vi "4.7.vi"() -> (0 "请在1-1000猜":dbl format="%#g", 1 "循环次数":i32, 2 "随机数":i32)   [LabVIEW 2017]
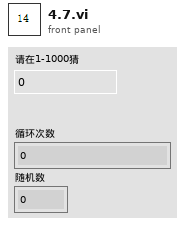
[diagram p1: front panel]
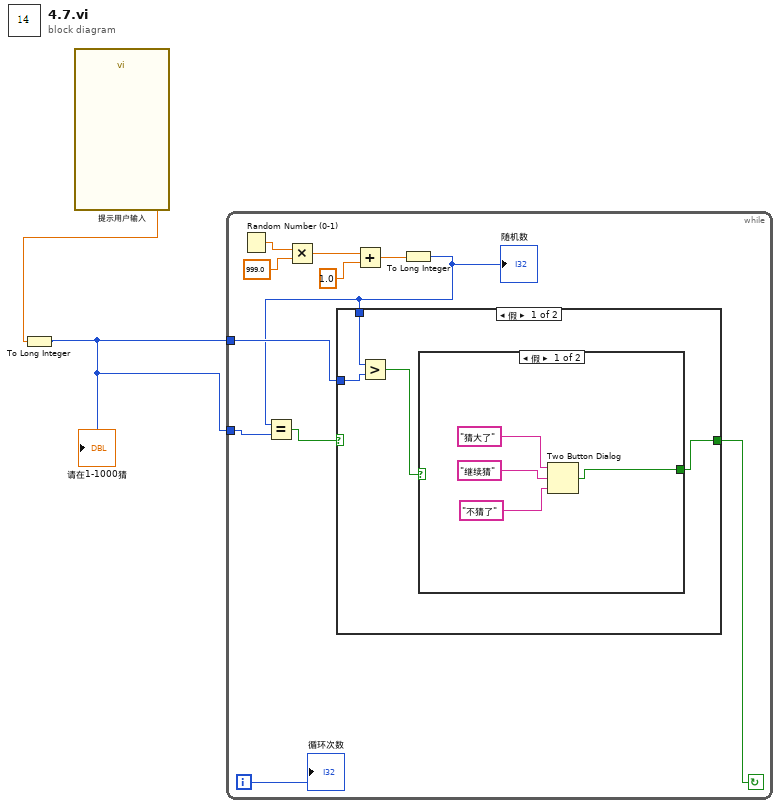
[diagram p0: block diagram]
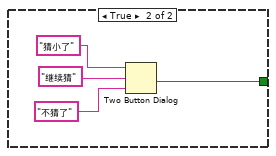
[diagram p2: hidden frame]
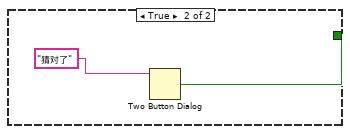
[diagram p3: hidden frame]
diagram:
  n1 = call "提示用户输入"() -> ("请在1-1000猜"=w2:dbl)  [unwired: 17 in, 2 out]
  n2 = To Long Integer(number=w2) -> (32bit integer=w1:i32)
  "请在1-1000猜" <- w1
  n3 = while {
    tunnel: w1 -> [w7]
    tunnel: w1 -> [w5]
    i -> [w9]
    stop <- w3 continue-if-true
    n4 = Random Number (0-1)() -> (number: 0 to 1=w13:dbl)
    n5 = Multiply(x=w13, y=999.0) -> (x*y=w11:dbl)
    n6 = Add(x=w11, y=1.0) -> (x+y=w8:dbl)
    n7 = To Long Integer(number=w8) -> (32bit integer=w4:i32)
    "随机数" <- w4
    n8 = Equal?(x=w4, y=w7) -> (x = y?=w6:bool)
    n9 = case shown="假" w6 {
      tunnel: w5 -> [w17 _]
      tunnel: w4 -> [w16 _]
      tunnel: [w14 w26] -> w3
      frame False {
        n10 = Greater?(x=w16, y=w17) -> (0:w15:bool)
        n11 = case shown="假" w15 {
          tunnel: [w20 w24] -> w14
          frame False {
            n12 = Two Button Dialog(message="猜大了", 1:"不猜了", 2:"继续猜") -> (T button?=w20:bool)
          }
          frame True {
            n13 = Two Button Dialog(message="猜小了", 1:"不猜了", 2:"继续猜") -> (T button?=w24:bool)
          }
        }
      }
      frame True {
        n14 = Two Button Dialog(message="猜对了") -> (T button?=w26:bool)  [unwired: 2 in]
      }
    }
    "循环次数" <- w9
  }
